vi "Main.vi"(8 "error in":errorcluster, 11 "ModuleB in":refnum<class "ModuleB.lvclass">) -> (0 "error out":errorcluster, 3 "ModuleB out":refnum<class "ModuleB.lvclass">)   [LabVIEW 2024, in "ModuleB.lvclass"]
doc: "The <b>Queued Message Handler</b> of the Worker that owns this VI."
uses:
  ModuleB.lvclass
  Initialization Data.ctl
  Response Cases.ctl
  <vilib>/addons/_Workers/Library/Case Label.ctl
  ModuleB.lvclass/ModuleB.ctl
  rql_ReadMeterValueProcess.ctl
  rwr_RequestMeterValue.ctl
  rwr_RequestMeterValue Reply.ctl
  3a1a03d0-d0fc-422f-9294-6291f42af5c2.vi
  <vilib>/addons/_Workers/Library/Workers.lvlib
panel:
  out "Progress":u8(slide) scale=0.0..100.0
  out "Meter":dbl(knob) scale=20.0..30.0
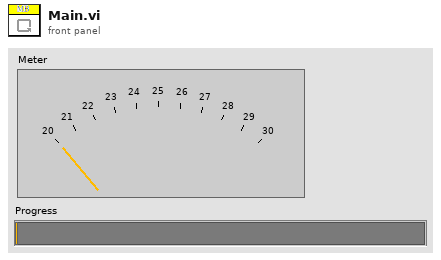
[diagram p1: front panel]
types:
  T1 = typedef "ModuleB.lvclass/Initialization Data.ctl" = cluster{"Response Cases":T2}
  T2 = typedef "ModuleB.lvclass/Response Cases.ctl" = cluster{"Placeholder - Can be deleted":string, "ReturnMeterValue":T3}
  T3 = typedef "Workers.lvlib/Case Label.ctl" = string
  T4 = typedef "ModuleB.lvclass/rql_ReadMeterValueProcess.ctl" = cluster{"String":string}
  T5 = typedef "ModuleB.lvclass/rwr_RequestMeterValue Reply.ctl" = cluster{"String":string, "MeterValue":dbl}
  T6 = typedef "ModuleB.lvclass/rwr_RequestMeterValue.ctl" = cluster{"String":string}
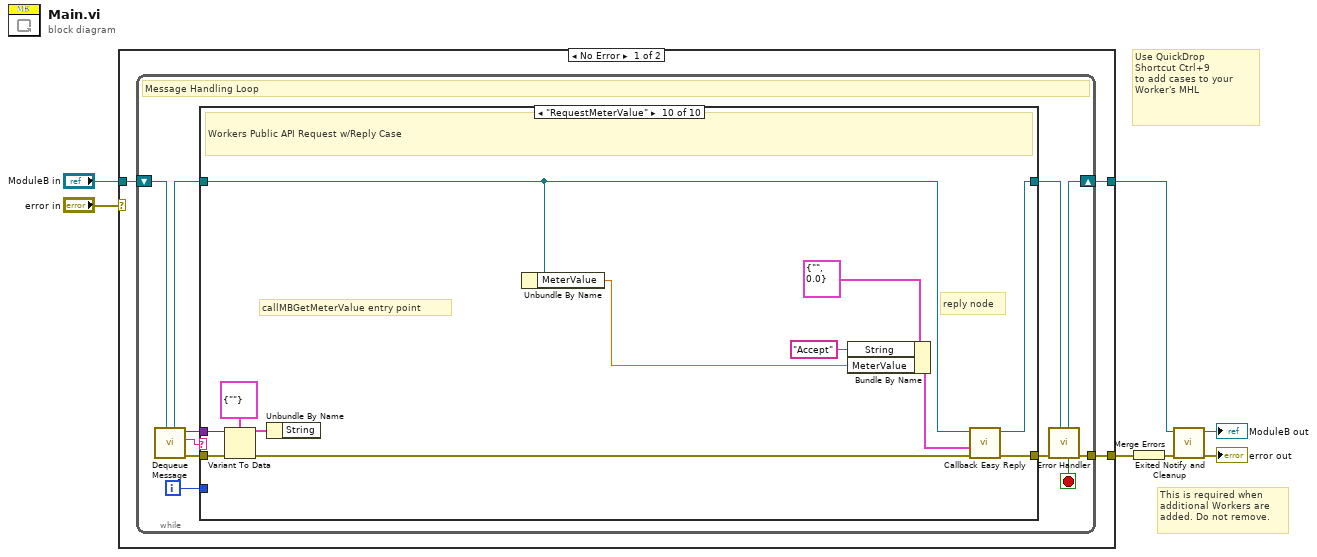
[diagram p0: block diagram]
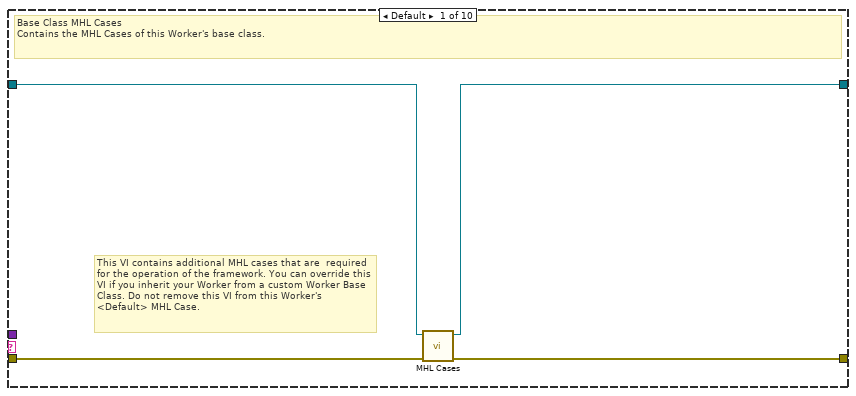
[diagram p2: hidden frame]
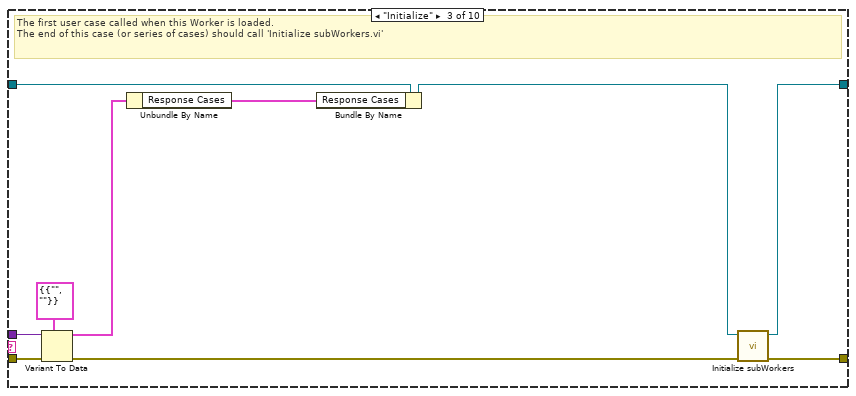
[diagram p4: hidden frame]
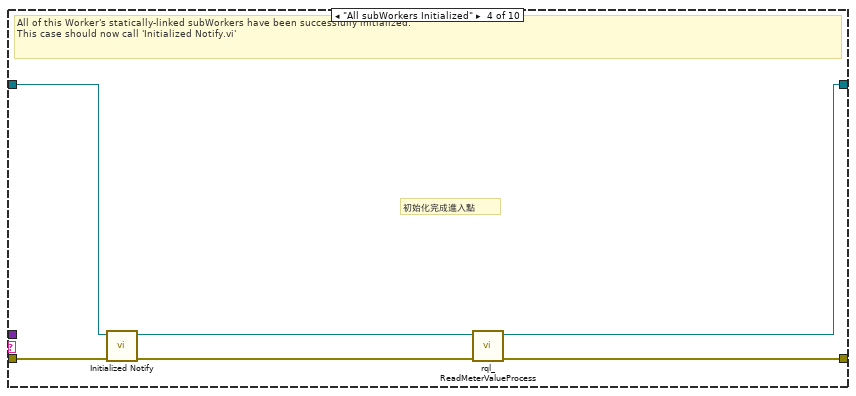
[diagram p5: hidden frame]
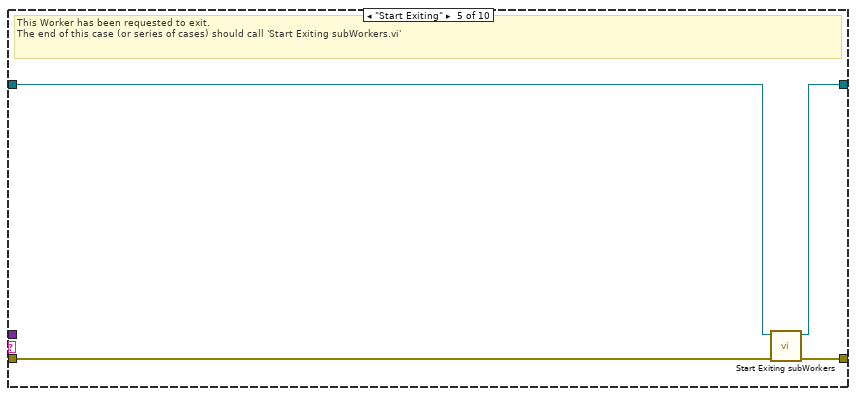
[diagram p6: hidden frame]
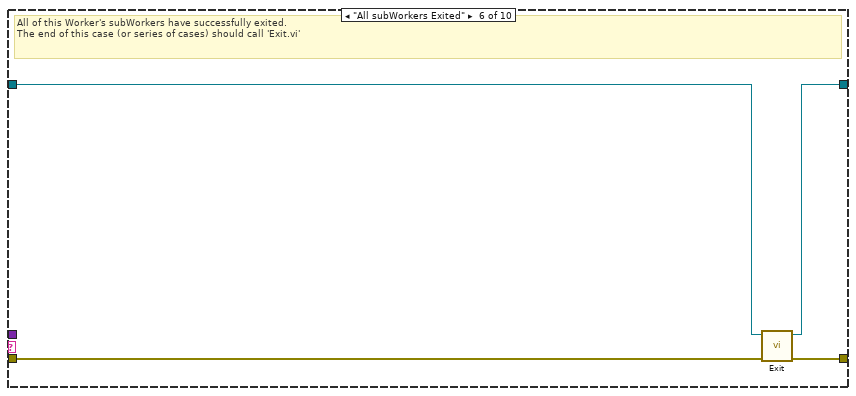
[diagram p7: hidden frame]
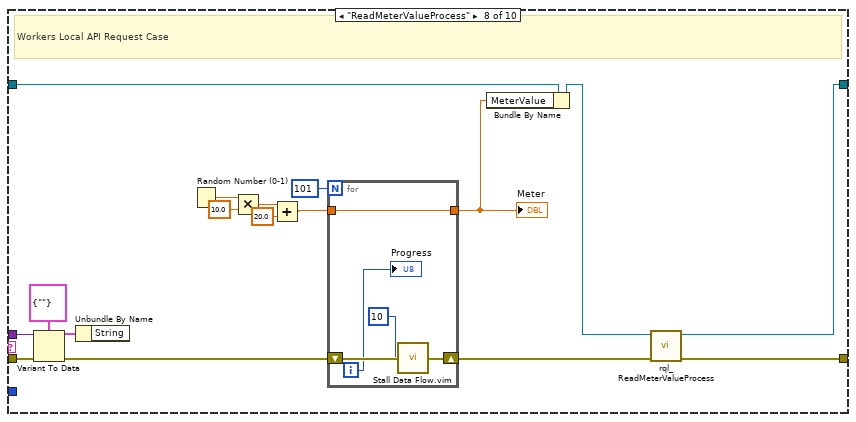
[diagram p9: hidden frame]
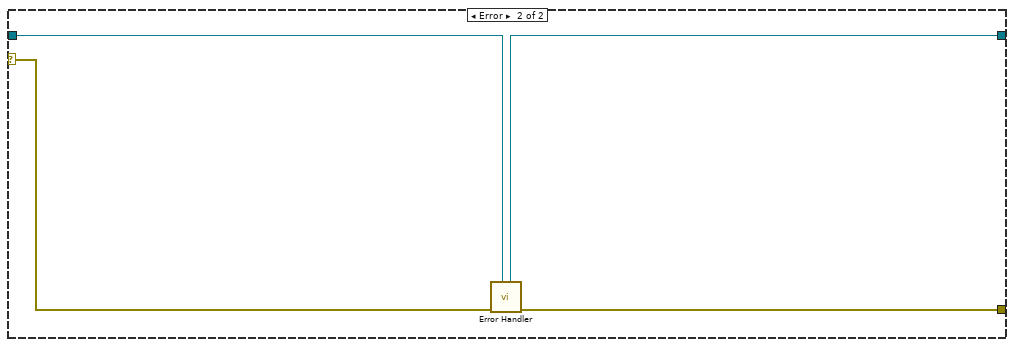
[diagram p11: hidden frame]
diagram:
  # "Use QuickDrop\nShortcut Ctrl+9\nto add cases to your\nWorker's MHL"
  # "This is required when additional Workers are added. Do not remove."
  n1 = case shown="No Error" "error in" {
    tunnel: "ModuleB in" -> [w8 w91]
    tunnel: [w10 w92] -> w6
    tunnel: [w9 w90] -> w7
    selector: "error in" -> [_ w93]
    frame No Error {
      n2 = while {
        shift-right: [w19] -> w9
        shift-left: w8 -> [w21]
        tunnel: [w20] -> w10
        i -> [w12]
        stop <- w13 stop-if-true
        # "Message Handling Loop"
        n3 = call-dynamic "Dequeue Message.vi"("Worker"=w21) -> ("error out"=w18:errorcluster, "Case out"=w14:string, "Data out"=w11:variant, "Worker out"=w16:refnum<class "ModuleB.lvclass">)  [unwired: 6 in, 1 out]
        n4 = case "Worker MHL Case Structure (DO NOT CHANGE LABEL NAME)" shown="\"RequestMeterValue\"" w14 {
          tunnel: w18 -> [w25 w26 w35 w43 w44 w51 w53 w70 w77 w89]
          tunnel: [w24 w26 w37 w40 w47 w50 w53 w58 w77 w84] -> w17
          tunnel: w16 -> [w23 w27 w34 w41 w45 w49 w52 w57 w76 w79]
          tunnel: [w22 w27 w36 w38 w46 w48 w52 w56 w76 w83] -> w15
          tunnel: w12 -> [_ _ _ _ _ _ _ _ _ _]
          tunnel: w11 -> [_ _ w32 _ _ _ _ w67 _ w86]
          frame Default {
            # "This VI contains additional MHL cases that are  required for the operation of the framework. You can override this VI if you inherit your Worker from a custom Worker Base Class. Do not remove this VI from this Worker's <Default> MHL Case."
            # "Base Class MHL Cases\nContains the MHL Cases of this Worker's base class."
            n5 = call-dynamic "MHL Cases.vi"("error in"=w25, "Worker in"=w23) -> ("error out"=w24:errorcluster, "Worker out"=w22:refnum<class "ModuleB.lvclass">)  [unwired: 8 in]
          }
          frame "------------ FRAMEWORK CASES -----------" {
            # "Start of Workers Framework Cases"
          }
          frame "Initialize" {
            # "The first user case called when this Worker is loaded.\nThe end of this case (or series of cases) should call 'Initialize subWorkers.vi'"
            n6 = Variant To Data(error in=w35, type=T1 {"Response Cases"={"Placeholder - Can be deleted"="", "ReturnMeterValue"=""}} ("Cluster"), Variant=w32) -> (data=w30:T1, error out=w33:errorcluster)
            n7 = Unbundle By Name(w30) -> ("Response Cases"=w29:T2)
            n8 = Bundle By Name(cluster=w34, "Response Cases"=w29) -> (w31:refnum<class "ModuleB.lvclass">)
            n9 = call-dynamic "Initialize subWorkers.vi"("error in"=w33, "Worker"=w31) -> ("error out"=w37:errorcluster, "dup Worker out"=w36:refnum<class "ModuleB.lvclass">)  [unwired: 8 in]
          }
          frame "All subWorkers Initialized" {
            # "初始化完成進入點"
            # "All of this Worker's statically-linked subWorkers have been successfully initialized.\nThis case should now call 'Initialized Notify.vi'"
            n10 = call-dynamic "Initialized Notify.vi"("error in"=w43, "Worker"=w41) -> ("error out"=w42:errorcluster, "dup Worker out"=w39:refnum<class "ModuleB.lvclass">)  [unwired: 8 in]
            n11 = call "rql_ReadMeterValueProcess.vi"("error in"=w42, "ModuleB in"=w39) -> ("error out"=w40:errorcluster, "dup ModuleB out"=w38:refnum<class "ModuleB.lvclass">)  [unwired: 8 in]
          }
          frame "Start Exiting" {
            # "This Worker has been requested to exit. \nThe end of this case (or series of cases) should call 'Start Exiting subWorkers.vi'"
            n12 = call-dynamic "Start Exiting subWorkers.vi"("error_in"=w44, "Worker"=w45) -> ("error out"=w47:errorcluster, "dup Worker out"=w46:refnum<class "ModuleB.lvclass">)  [unwired: 8 in]
          }
          frame "All subWorkers Exited" {
            # "All of this Worker's subWorkers have successfully exited. \nThe end of this case (or series of cases) should call 'Exit.vi'"
            n13 = call-dynamic "Exit.vi"("error_in"=w51, "Worker"=w49) -> ("error out"=w50:errorcluster, "dup Worker out"=w48:refnum<class "ModuleB.lvclass">)  [unwired: 8 in]
          }
          frame "------------- LOCAL API CASES -------------" {
            # "Start of Workers Local API Cases"
          }
          frame "ReadMeterValueProcess" {
            # "Workers Local API Request Case"
            n14 = Variant To Data(error in=w70, type=T4 {"String"=""} ("Data"), Variant=w67) -> (data=w66:T4, error out=w69:errorcluster)
            n15 = Unbundle By Name(w66) -> ()  [unwired: 1 out]
            n16 = Random Number (0-1)() -> (number: 0 to 1=w65:dbl)
            n17 = Multiply(x=w65, y=10.0) -> (x*y=w63:dbl)
            n18 = Add(x=w63, y=20.0) -> (x+y=w60:dbl)
            n19 = for {
              N: 101 -> [_]
              shift-right: [w74] -> w61
              shift-left: w69 -> [w75]
              tunnel: [w72] -> w54
              tunnel: w60 -> [w72]
              i -> [w71]
              n20 = call "Stall Data Flow.vim"("value in"=w75, "milliseconds to wait"=u32 10) -> ("value out"=w74:errorcluster)  [unwired: 1 out]
              "Progress" <- w71
            }
            "Meter" <- w54
            n21 = Bundle By Name(cluster=w57, "MeterValue"=w54) -> (w55:refnum<class "ModuleB.lvclass">)
            n22 = call "rql_ReadMeterValueProcess.vi"("error in"=w61, "ModuleB in"=w55) -> ("error out"=w58:errorcluster, "dup ModuleB out"=w56:refnum<class "ModuleB.lvclass">)  [unwired: 8 in]
          }
          frame "------------- PUBLIC API CASES -------------" {
            # "Start of Workers Public API Cases"
          }
          frame "RequestMeterValue" {
            # "callMBGetMeterValue entry point"
            # "reply node"
            # "Workers Public API Request w/Reply Case"
            n23 = Variant To Data(error in=w89, type=T6 {"String"=""} ("Data"), Variant=w86) -> (data=w85:T6, error out=w88:errorcluster)
            n24 = Unbundle By Name(w85) -> ()  [unwired: 1 out]
            n25 = Unbundle By Name(w79) -> ("MeterValue"=w78:dbl)
            n26 = Bundle By Name(cluster=T5 {"String"="", "MeterValue"=0.0} ("Reply Data"), "String"="Accept", "MeterValue"=w78) -> (w81:T5)
            n27 = call-dynamic "Callback Easy Reply.vi"("error in"=w88, "Data"=w81, "Worker"=w79) -> ("error out"=w84:errorcluster, "dup Worker out"=w83:refnum<class "ModuleB.lvclass">)  [unwired: 7 in]
          }
        }
        n28 = call-dynamic "Error Handler.vi"("Worker"=w15, "error_in"=w17) -> ("error out"=w20:errorcluster, "Stop Loop"=w13:bool, "Worker out"=w19:refnum<class "ModuleB.lvclass">)  [unwired: 7 in]
      }
    }
    frame Error {
      n29 = call-dynamic "Error Handler.vi"("Worker"=w91, "error_in"=w93) -> ("error out"=w92:errorcluster, "Worker out"=w90:refnum<class "ModuleB.lvclass">)  [unwired: 7 in, 1 out]
    }
  }
  n30 = Merge Errors(w6) -> (w3:errorcluster)
  n31 = call-dynamic "Exited Notify and Cleanup.vi"("error_in"=w3, "Worker"=w7) -> ("error out"=→"error out":errorcluster, "dup Worker out"=→"ModuleB out":refnum<class "ModuleB.lvclass">)  [unwired: 8 in]
